vi "FiberSpectrograph_putSample_timestamp.vi"(8 "error in (no error)":errorcluster, 11 "timestamp_Ctl":T1) -> (0 "error out":errorcluster, 2 "function return":i32, 3 "timestamp_Ctl out":T1)   [LabVIEW 2016, in "SALLV_FiberSpectrograph.lvlib"]
doc: "int FiberSpectrograph_shm_putSample_timestampLV(FiberSpectrograph_timestampLV *timestamp_Ctl );"
uses:
  SALLV_FiberSpectrograph.lvlib
  DataTypes/timestamp.ctl
  SALLV_FiberSpectrograph.so
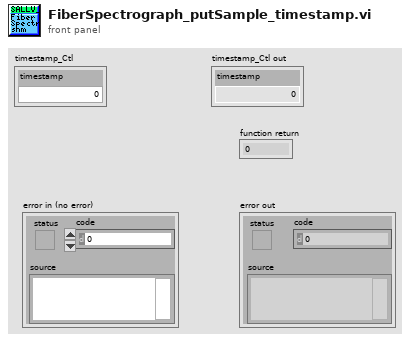
[diagram p1: front panel]
types:
  T1 = typedef "SALLV_FiberSpectrograph.lvlib/timestamp.ctl" = cluster{"timestamp":dbl}
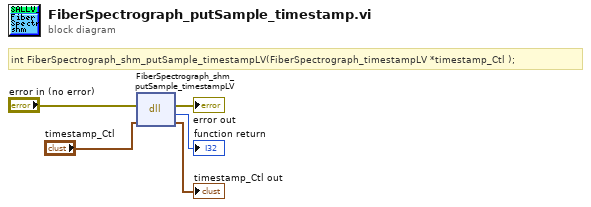
[diagram p0: block diagram]
diagram:
  # "int FiberSpectrograph_shm_putSample_timestampLV(FiberSpectrograph_timestampLV *timestamp_Ctl );"
  n1 = dll-call lib="home/harini/tcs/temp/SALLV_FiberSpectrograph.*" fn="FiberSpectrograph_shm_putSample_timestampLV"(error in="error in (no error)", "timestamp_Ctl"="timestamp_Ctl") -> (error out=→"error out":errorcluster, →"function return":i32, "timestamp_Ctl"=→"timestamp_Ctl out":T1)  [unwired: 2 in, 1 out]
